vi "jsq_test.vi"() -> ()   [LabVIEW 2015, in "oskar_tools.lvlib"]
uses:
  oskar_tools.lvlib
  seq_line.ctl
panel:
  out "pretty print":string
  out "JSON string":string
  out "SEQs":T1[](array[typedef])
  in  "Open":path=path "C:/Users/Adam/Desktop/test.osq"
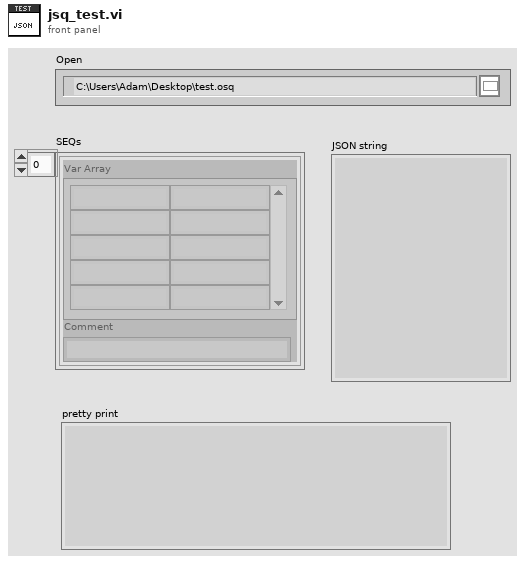
[diagram p1: front panel]
types:
  T1 = typedef "oskar_tools.lvlib/seq_line.ctl" = cluster{"Var Array":string[][], "Comment":string}
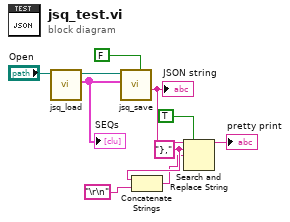
[diagram p0: block diagram]
diagram:
  w5 = "}," ("search string")
  n1 = call "jsq_load.vi"("Open"="Open") -> ("SEQs"=w9:T1[], "json file path(duplicate)"=w8:path)  [unwired: 7 in, 2 out]
  "SEQs" <- w9
  n2 = call "jsq_save.vi"("Save?"=FALSE, "SEQs"=w9, "Path"=w8) -> ("JSON string"=w6:string)  [unwired: 6 in, 2 out]
  "JSON string" <- w6
  n3 = Concatenate Strings(w5, "\r\n") -> (w4:string)
  n4 = Search and Replace String(replace all?=TRUE ("replace all? (F)"), input string=w6, search string=w5, replace string=w4) -> (result string=→"pretty print":string)  [unwired: 4 in, 3 out]
